vi "Write EventData.vi"(8 "error in (no error)":errorcluster, 10 "EventData":cluster{"Classification":T1}, 11 "Event in":refnum<class "Event.lvclass">) -> (0 "error out":errorcluster, 3 "Event out":refnum<class "Event.lvclass">)   [LabVIEW 2019, in "Event.lvclass"]
uses:
  Event.lvclass
  TypeDef/Event Classification.ctl
  Event.lvclass/Event.ctl
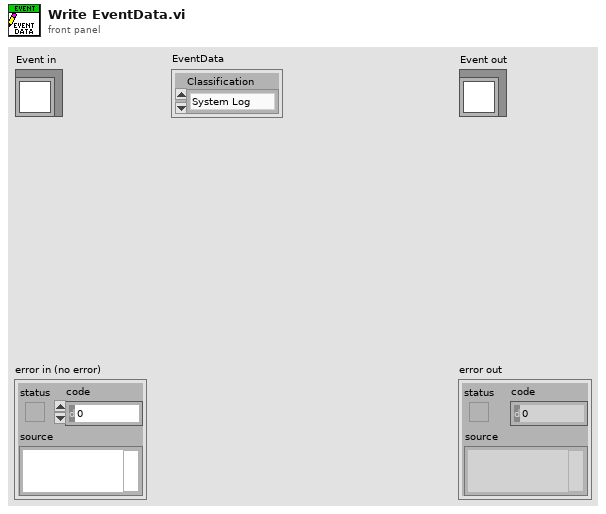
[diagram p1: front panel]
types:
  T1 = typedef "Event.lvclass/Event Classification.ctl" = enum16{"System Log"}
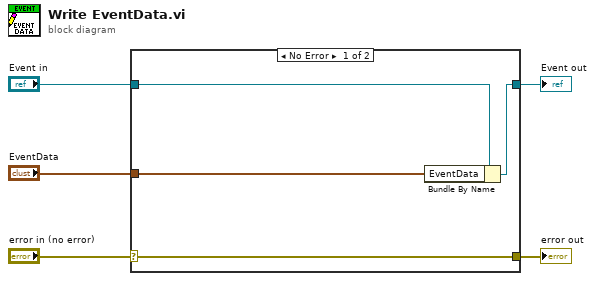
[diagram p0: block diagram]
diagram:
  n1 = case shown="No Error" "error in (no error)" {
    selector: "error in (no error)" -> [w9 w10]
    tunnel: [w9 w10] -> w4
    tunnel: [w7 w11] -> w2
    tunnel: "Event in" -> [w8 w11]
    tunnel: "EventData" -> [w6 _]
    frame No Error {
      n2 = Bundle By Name(cluster=w8, "EventData"=w6) -> (w7:refnum<class "Event.lvclass">)
    }
    frame Error {
    }
  }
  "error out" <- w4
  "Event out" <- w2
